vi "dosimat876.vi"() -> ()   [LabVIEW 2010]
panel:
  in  "Check volume":bool
  out "Volume":dbl
  out "error out":errorcluster
  out "Coerced?":bool
  in  "Dosimat Port":refnum<visa-resource-name>="COM10"
  in  "stop":bool=TRUE
  out "Total Volume\nDelivered":dbl format="%.3f"
  in  "Zero Volume":bool
  in  "Volume to be\nDelivered":dbl=0.05 format="%.3f"
  in  "Fill Burette":bool
  in  "Dispense Volume":bool
  # "Volume coerced!\nThe 876 will only accept volumes between 0.05 and 5.00 ml in increments of 0.05 ml. The volume has been changed to meet these requirements."
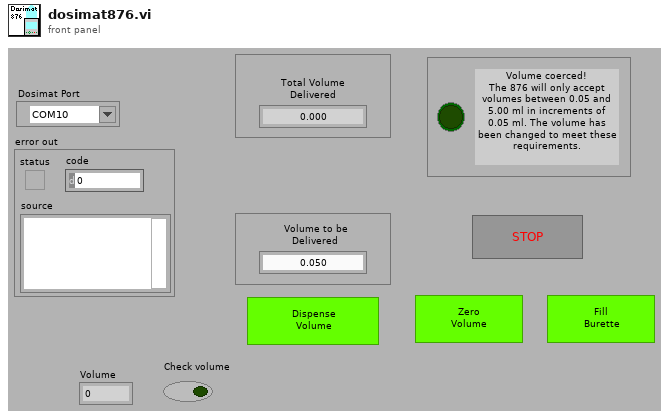
[diagram p1: front panel]
types:
  T1 = cluster{"Dosimat Port out":refnum<visa-resource-name>, "Error out":errorcluster}
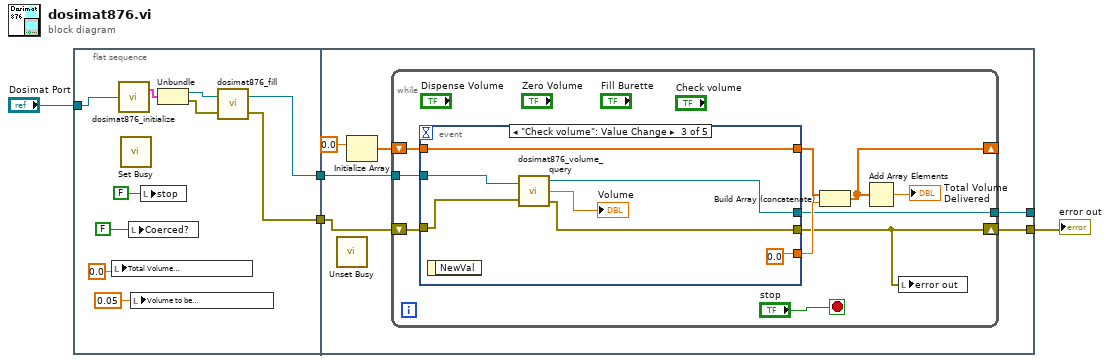
[diagram p0: block diagram]
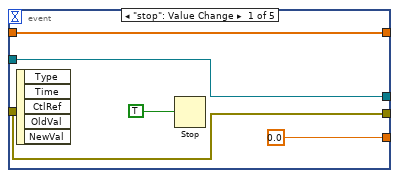
[diagram p2: hidden frame]
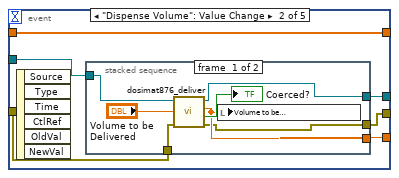
[diagram p3: hidden frame]
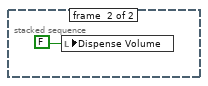
[diagram p4: hidden frame]
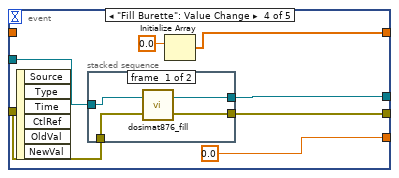
[diagram p5: hidden frame]
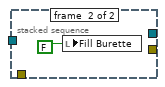
[diagram p6: hidden frame]
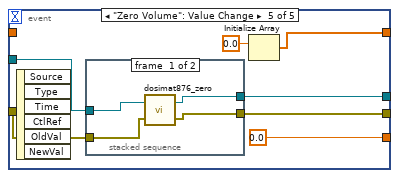
[diagram p7: hidden frame]
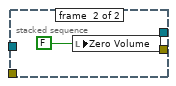
[diagram p8: hidden frame]
diagram:
  n1 = flat-sequence {
    tunnel: "Dosimat Port" -> [w10]
    tunnel: [w9] -> w3
    tunnel: [w8] -> w2
    tunnel: w3 -> [w20]
    tunnel: w2 -> [w17]
    tunnel: [w16] -> _
    tunnel: [w15] -> w1
    frame #0 {
      n2 = local write "Total Volume\nDelivered"(0.0 ("Total Volume\nDelivered")) -> ()
      n3 = call "dosimat876_initialize.vi"("Dosimat Port In"=w10) -> ("Dosimat Out"=w7:T1)  [unwired: 1 in]
      n4 = call <vilib>:"Set Busy.vi"() -> ()  [unwired: 10 in, 2 out]
      n5 = local write "Coerced?"(FALSE ("stop")) -> ()
      n6 = local write "Volume to be\nDelivered"(0.05 ("Volume to be\nDelivered")) -> ()
      n7 = local write "stop"(FALSE ("stop")) -> ()
      n8 = Unbundle(w7) -> ("Dosimat Port out"=w6:refnum<visa-resource-name>, "Error out"=w5:errorcluster)
      n9 = call "dosimat876_fill.vi"("error in"=w5, "Dosimat Port In"=w6) -> ("error out"=w8:errorcluster, "Dosimat Port Out"=w9:refnum<visa-resource-name>)
    }
    frame #1 {
      n10 = call <vilib>:"Unset Busy.vi"() -> ()  [unwired: 11 in, 1 out]
      n11 = Initialize Array(0.0 ("element")) -> (w18:dbl[])  [unwired: 1 in]
      n12 = while {
        tunnel: w20 -> [w30]
        shift-right: [w26] -> _
        shift-left: w18 -> [w25]
        tunnel: [w22] -> w16
        shift-right: [w21] -> w15
        shift-left: w17 -> [w23]
        stop <- "stop" stop-if-true
        n13 = event shown="[2] \"Check volume\": Value Change" {
          selector: _ -> [_ _ _ _ _]
          dyn-events: _ -> [_ _ _ _ _]
          timeout: _ -> [_ _ _ _ _]
          tunnel: w30 -> [w31 w41 w56 w63 w75]
          tunnel: [0.0 ("Volume to be\nDelivered") w40 0.0 0.0 ("Volume to be\nDelivered") 0.0 ("Volume to be\nDelivered")] -> w27
          tunnel: w25 -> [w33 w39 w50 _ _]
          tunnel: [w33 w39 w50 w60 w72] -> w24
          tunnel: w23 -> [w32 w38 w53 w59 w71]
          tunnel: [w31 w37 w55 w58 w69] -> w22
          tunnel: [w32 w36 w54 w57 w70] -> w21
          event "stop": Value Change {
            n14 = event-data() -> ()  [unwired: 1 in, 5 out]
            n15 = Stop(stop? (T)=TRUE ("stop")) -> ()
          }
          event "Dispense Volume": Value Change {
            n16 = event-data() -> ()  [unwired: 1 in, 6 out]
            n17 = stacked-sequence {
              tunnel: w41 -> [w48 _]
              tunnel: [w45 _] -> w40
              tunnel: w38 -> [w44 _]
              tunnel: [w43 _] -> w37
              tunnel: [w42 _] -> w36
              frame #0 {
                n18 = call "dosimat876_deliver.vi"("error in"=w44, "Volume"="Volume to be\nDelivered", "Dosimat Port In"=w48) -> ("error out"=w42:errorcluster, "Coerced?"=→"Coerced?":bool, "OutVolume"=w45:dbl, "Dosimat Port Out"=w43:refnum<visa-resource-name>)  [unwired: 1 in]
                n19 = local write "Volume to be\nDelivered"(w45) -> ()
              }
              frame #1 {
                n20 = local write "Dispense Volume"(FALSE) -> ()
              }
            }
          }
          event "Check volume": Value Change {
            n21 = event-data() -> ()  [unwired: 1 in, 1 out]
            n22 = call "dosimat876_volume_query.vi"("error in"=w53, "Dosimat Port In"=w56) -> ("error out"=w54:errorcluster, "Volume"=→"Volume":dbl, "Dosimat Port Out"=w55:refnum<visa-resource-name>)
          }
          event "Fill Burette": Value Change {
            n23 = event-data() -> ()  [unwired: 1 in, 6 out]
            n24 = stacked-sequence {
              tunnel: w63 -> [w67 _]
              tunnel: w59 -> [w66 _]
              tunnel: [w65 _] -> w58
              tunnel: [w64 _] -> w57
              frame #0 {
                n25 = call "dosimat876_fill.vi"("error in"=w66, "Dosimat Port In"=w67) -> ("error out"=w64:errorcluster, "Dosimat Port Out"=w65:refnum<visa-resource-name>)
              }
              frame #1 {
                n26 = local write "Fill Burette"(FALSE) -> ()
              }
            }
            n27 = Initialize Array(0.0 ("element")) -> (w60:dbl[])  [unwired: 1 in]
          }
          event "Zero Volume": Value Change {
            n28 = event-data() -> ()  [unwired: 1 in, 6 out]
            n29 = stacked-sequence {
              tunnel: w75 -> [w79 _]
              tunnel: w71 -> [w78 _]
              tunnel: [w77 _] -> w70
              tunnel: [w76 _] -> w69
              frame #0 {
                n30 = call "dosimat876_zero.vi"("error in"=w78, "Dosimat Port In"=w79) -> ("error out"=w77:errorcluster, "Dosimat Port Out"=w76:refnum<visa-resource-name>)
              }
              frame #1 {
                n31 = local write "Zero Volume"(FALSE) -> ()
              }
            }
            n32 = Initialize Array(0.0 ("element")) -> (w72:dbl[])  [unwired: 1 in]
          }
        }
        n33 = Build Array (concatenate)(w24, w27) -> (w26:dbl[])
        n34 = Add Array Elements(numeric array=w26) -> (sum=→"Total Volume\nDelivered":dbl)
        n35 = local write "error out"(w21) -> ()
      }
    }
  }
  "error out" <- w1
